vi "Set Steering Wheel Parameters.vi"(8 "error in (no error)":errorcluster, 10 "steering parameters":T1={"steering gear ratio"=1.0, "motor angle offset (rad)"=0.0, "steering angle range"={"min steering angle (rad)"=-3.14159, "max steering angle (rad)"=3.141592653589793}}, 11 "steering wheel in":refnum<class "NI_Robotics_Steering Wheel.lvclass">) -> (0 "error out":errorcluster, 3 "steering wheel out":refnum<class "NI_Robotics_Steering Wheel.lvclass">)   [LabVIEW 2017, in "NI_Robotics_Steering Wheel.lvclass"]
uses:
  <vilib>/robotics/Steering/Steering Wheel/NI_Robotics_Steering Wheel.lvclass
  <vilib>/robotics/Steering/Steering Wheel/Steering Wheel Parameters.ctl
  <vilib>/robotics/Steering/Steering Wheel/Steering Angle Range.ctl
  <vilib>/robotics/Steering/Steering Wheel/NI_Robotics_Steering Wheel.lvclass/NI_Robotics_Steering Wheel.ctl
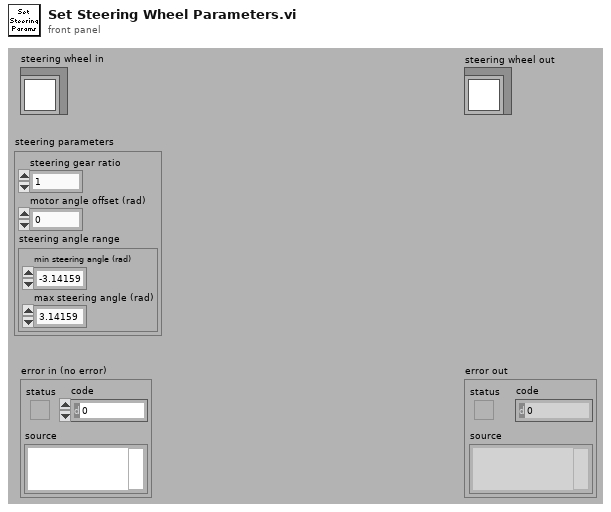
[diagram p1: front panel]
types:
  T1 = typedef "NI_Robotics_Steering Wheel.lvclass/Steering Wheel Parameters.ctl" = cluster{"steering gear ratio":dbl, "motor angle offset (rad)":dbl, "steering angle range":T2}
  T2 = typedef "NI_Robotics_Steering Wheel.lvclass/Steering Angle Range.ctl" = cluster{"min steering angle (rad)":dbl, "max steering angle (rad)":dbl}
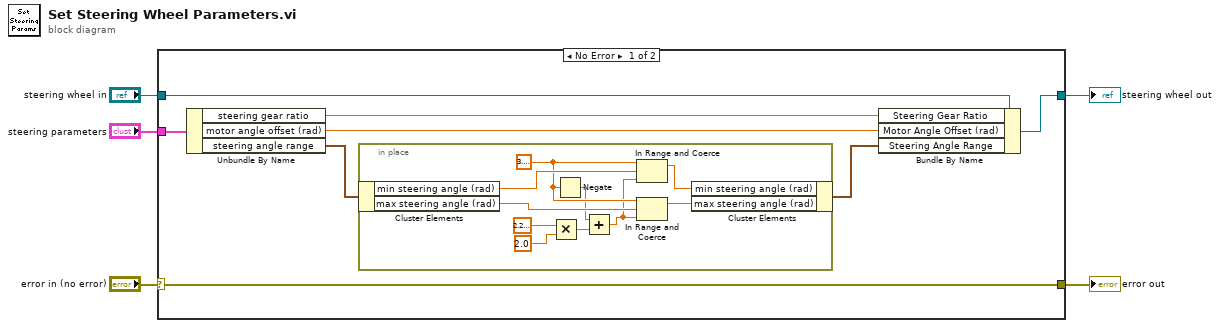
[diagram p0: block diagram]
diagram:
  n1 = case shown="No Error" "error in (no error)" {
    selector: "error in (no error)" -> [w13 w25]
    tunnel: [w13 w25] -> w4
    tunnel: [w10 w24] -> w2
    tunnel: "steering wheel in" -> [w11 w24]
    tunnel: "steering parameters" -> [w12 _]
    frame No Error {
      n2 = Unbundle By Name(w12) -> ("steering gear ratio"=w9:dbl, "motor angle offset (rad)"=w8:dbl, "steering angle range"=w7:T2)
      n3 = in-place {
        w19 = 3.141592653589793
        n4 = in-place-cluster #1(w7) -> ("min steering angle (rad)"=w23:dbl, "max steering angle (rad)"=w21:dbl)
        n5 = Multiply(x=2.220446049250313e-16, y=2.0) -> (x*y=w16:dbl)
        n6 = Negate(x=w19) -> (-x=w15:dbl)
        n7 = Add(x=w15, y=w16) -> (x+y=w14:dbl)
        n8 = In Range and Coerce(upper limit=w19, x=w23, lower limit=w14) -> (coerced(x)=w22:dbl)  [unwired: 1 out]
        n9 = In Range and Coerce(upper limit=w19, x=w21, lower limit=w14) -> (coerced(x)=w20:dbl)  [unwired: 1 out]
        n10 = in-place-cluster #1("min steering angle (rad)"=w22, "max steering angle (rad)"=w20) -> (w6:T2)
      }
      n11 = Bundle By Name(cluster=w11, "Steering Gear Ratio"=w9, "Motor Angle Offset (rad)"=w8, "Steering Angle Range"=w6) -> (w10:refnum<class "NI_Robotics_Steering Wheel.lvclass">)
    }
    frame Error {
    }
  }
  "error out" <- w4
  "steering wheel out" <- w2
